vi "Test Drive Inputs.vi"   [LabVIEW 2017]
uses:
  GitHub/RamonaRampage/Development/Dev1/Support Code/Globals/Reference Names Global.vi
types:
  T1 = typedef "Joystick Controls.ctl" = cluster{"Joystick Left - Right":dbl, "Joystick Up-Down":dbl, "Joystick Twist":dbl, "Joystick Throttle":dbl, "Joystick Trigger":bool, "Joystick Thumb Button":bool, "Joystick Button 3":bool, "Joystick Button 4":bool, "Joystick Button 5":bool, "Joystick Button 6":bool, "Joystick Button 7":bool, "Joystick Button 8":bool, "Joystick Button 9":bool, "Joystick Button 10":bool, "Joystick Button 11":bool, "Joystick Button 12":bool, "POV":i16, "POV 2":i16}
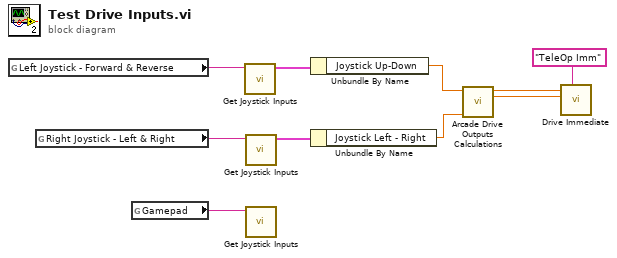
[diagram p0: block diagram]
diagram:
  n1 = global read "Reference Names Global.vi" "Left Joystick - Forward & Reverse"() -> (w8:string)
  n2 = global read "Reference Names Global.vi" "Right Joystick - Left & Right"() -> (w10:string)
  n3 = global read "Reference Names Global.vi" "Gamepad"() -> (w9:string)
  n4 = call "Get Joystick Inputs.vi"("Joystick Refnum"=w8) -> ("Joystick Output"=w7:T1)  [unwired: 10 in]
  n5 = call "Get Joystick Inputs.vi"("Joystick Refnum"=w10) -> ("Joystick Output"=w6:T1)  [unwired: 10 in]
  n6 = call "Get Joystick Inputs.vi"("Joystick Refnum"=w9) -> ()  [unwired: 10 in, 1 out]
  n7 = Unbundle By Name(w7) -> ("Joystick Up-Down"=w5:dbl)
  n8 = Unbundle By Name(w6) -> ("Joystick Left - Right"=w2:dbl)
  n9 = call "Arcade Drive Outputs Calculations.vi"("Turning Left & Right (Right Joystick)"=w2, "Speed Forward & Reverse (Left JoysticK)"=w5) -> ("Right Motor"=w1:dbl, "Left Motor"=w3:dbl)  [unwired: 8 in]
  n10 = call "Drive Immediate.vi"("Description"="TeleOp Imm", "Right Setpoint"=w1, "Left Setpoint"=w3) -> ()  [unwired: 8 in, 1 out]
